vi "Configure SoftCal.vi"(0 "VISA resource name":refnum<visa-resource-name>, 1 "First Temperature Point (4.2000)":dbl=4.2 min=2.0 max=100.0 step=0.0001 format="%.4f", 2 "Second Temperature Point (77.3500)":dbl=77.35 min=50.0 max=325.0 step=0.0001 format="%.4f", 3 "Third Temperature Point (305.0000)":dbl=305.0 min=200.0 max=600.0 step=0.0001 format="%.4f", 5 "Standard Curve (0: DT-470)":u16(ring) items=["DT-470", "PT-100", "PT-1000"], 7 "User Curve(21)":dbl=21.0 min=21.0 max=41.0 step=1.0, 9 "Serial Number (\"\")":string, 11 "error in (no error)":errorcluster, 12 "First Sensor Units Point (1.62622)":dbl=1.62622 min=1e-05 max=9999.99999 step=1e-05 format="%.5f", 13 "Second Sensor Units Point (1.02032)":dbl=1.02032 min=1e-05 max=9999.99999 step=1e-05 format="%.5f", 14 "Third Sensor Units Point (0.50691)":dbl=0.50691 min=1e-05 max=9999.99999 step=1e-05 format="%.5f") -> (4 "VISA resource name out":refnum<visa-resource-name>, 15 "error out":errorcluster)   [LabVIEW 2013, in "Lake Shore Cryotronics 331.lvlib"]
doc: "This VI generates a SoftCal curve from a standard curve and saves it in one of the user curve locations. Standard curves available for SoftCal generation are DT-470, PT-100, and PT-1000."
uses:
  Lake Shore Cryotronics 331.lvlib
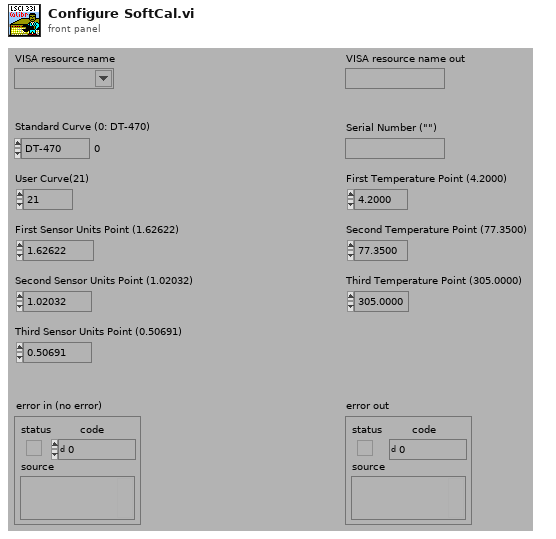
[diagram p1: front panel]
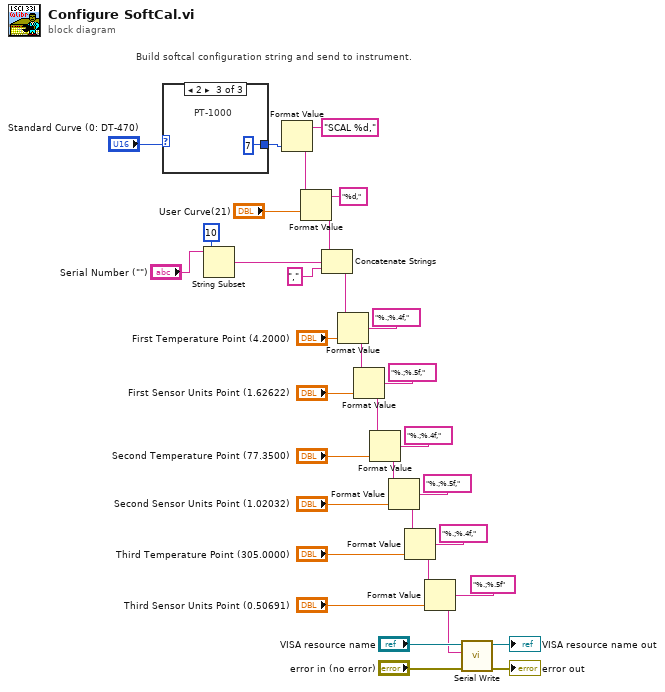
[diagram p0: block diagram]
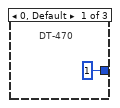
[diagram p2: hidden frame]
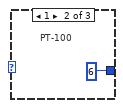
[diagram p3: hidden frame]
diagram:
  # "Build softcal configuration string and send to instrument."
  n1 = case shown="2" "Standard Curve (0: DT-470)" {
    tunnel: [1 6 7] -> w1
    frame 0, Default {
      # "DT-470"
    }
    frame 1 {
      # "PT-100"
    }
    frame 2 {
      # "PT-1000"
    }
  }
  n2 = String Subset(string="Serial Number (\"\")", length (rest)=10) -> (substring=w33:string)  [unwired: 1 in]
  n3 = Format Value(format string="SCAL %d,", value (0)=w1) -> (output string=w27:string)  [unwired: 1 in]
  n4 = Format Value(string ("")=w27, format string="%d,", value (0)="User Curve(21)") -> (output string=w26:string)
  n5 = Concatenate Strings(w26, w33, ",") -> (w24:string)
  n6 = Format Value(string ("")=w24, format string="%.;%.4f,", value (0)="First Temperature Point (4.2000)") -> (output string=w3:string)
  n7 = Format Value(string ("")=w3, format string="%.;%.5f,", value (0)="First Sensor Units Point (1.62622)") -> (output string=w19:string)
  n8 = Format Value(string ("")=w19, format string="%.;%.4f,", value (0)="Second Temperature Point (77.3500)") -> (output string=w16:string)
  n9 = Format Value(string ("")=w16, format string="%.;%.5f,", value (0)="Second Sensor Units Point (1.02032)") -> (output string=w13:string)
  n10 = Format Value(string ("")=w13, format string="%.;%.4f,", value (0)="Third Temperature Point (305.0000)") -> (output string=w10:string)
  n11 = Format Value(string ("")=w10, format string="%.;%.5f", value (0)="Third Sensor Units Point (0.50691)") -> (output string=w4:string)
  n12 = call "Serial Write.vi"("error in (no error)"="error in (no error)", "Write Buffer (\"\")"=w4, "VISA resource name"="VISA resource name") -> ("error out"=→"error out":errorcluster, "VISA resource name out"=→"VISA resource name out":refnum<visa-resource-name>)  [unwired: 6 in, 1 out]
